vi "Write Group.vi"(8 "error in (no error)":errorcluster, 10 "Group":string, 11 "Update CVT Data in":refnum<class "Update CVT Data.lvclass">) -> (0 "error out":errorcluster, 3 "Update CVT Data out":refnum<class "Update CVT Data.lvclass">)   [LabVIEW 2014, in "Update CVT Data.lvclass"]
uses:
  Update CVT Data.lvclass
  Update CVT Data.lvclass/Update CVT Data.ctl
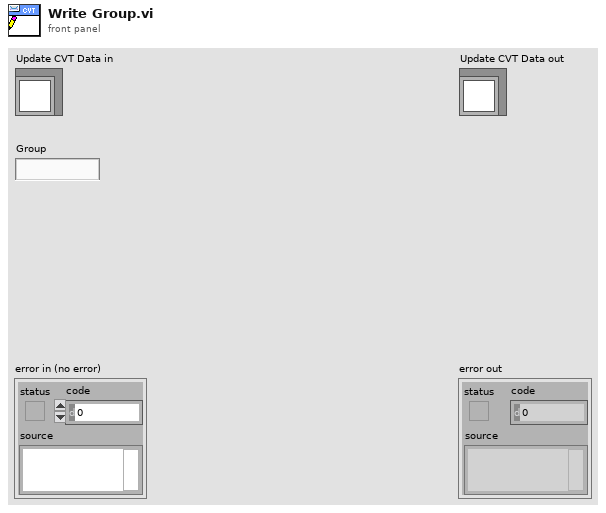
[diagram p1: front panel]
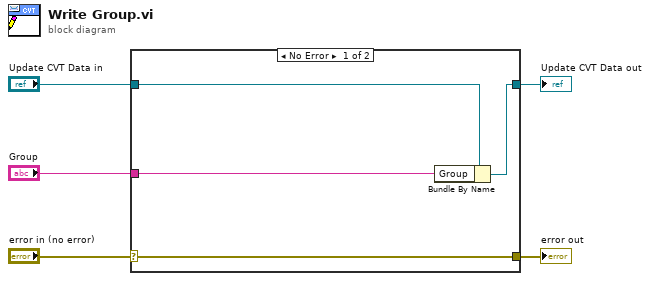
[diagram p0: block diagram]
diagram:
  n1 = case shown="No Error" "error in (no error)" {
    selector: "error in (no error)" -> [w9 w10]
    tunnel: [w9 w10] -> w4
    tunnel: [w7 w11] -> w2
    tunnel: "Update CVT Data in" -> [w8 w11]
    tunnel: "Group" -> [w6 _]
    frame No Error {
      n2 = Bundle By Name(cluster=w8, "Group"=w6) -> (w7:refnum<class "Update CVT Data.lvclass">)
    }
    frame Error {
    }
  }
  "error out" <- w4
  "Update CVT Data out" <- w2
